vi "move picture.vi"(0 "Picture in":picture, 3 "move":cluster{"x":i16, "y":i16}) -> (14 "Picture out":picture)   [LabVIEW 2019]
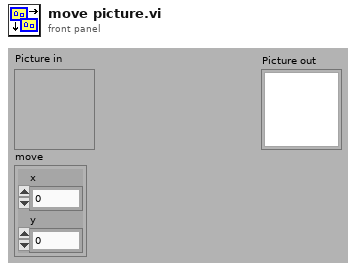
[diagram p1: front panel]
types:
  T1 = typedef "picture op-code.ctl" = u16
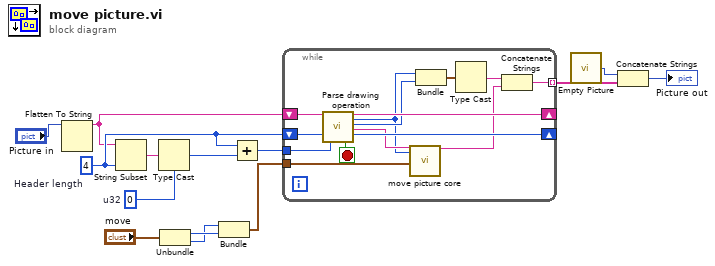
[diagram p0: block diagram]
diagram:
  w5 = u32 0  # u32
  w13 = 4  # Header length
  n1 = Flatten To String(anything="Picture in") -> (data string=w7:string)  [unwired: 3 in, 2 out]
  n2 = String Subset(string=w7, length (rest)=w13) -> (substring=w6:string)  [unwired: 1 in]
  n3 = Type Cast(type=w5, x=w6) -> (*(type *) &x=w14:u32)
  n4 = Unbundle("move") -> ("x"=w3:i16, "y"=w2:i16)
  n5 = Bundle("y"=w2, "x"=w3) -> (w1:cluster{"y":i16, "x":i16})  [unwired: 1 in]
  n6 = Add(x=w13, y=w14) -> (x+y=w12:u32)
  n7 = while {
    shift-right: [w23] -> _
    shift-left: w7 -> [w27]
    shift-right: [w26] -> _
    shift-left: w13 -> [w28]
    tunnel: w12 -> [w24]
    tunnel: [w18] -> w9 mode=indexing
    tunnel: w1 -> [w15]
    stop <- w25 stop-if-true
    n8 = call "Parse drawing operation.vi"("picture data in"=w27, "offset"=w28, "picture size"=w24) -> ("last element"=w25:bool, "picture data out"=w23:string, "op-code"=w16:T1, "data length"=w22:u32, "data string"=w17:string, "offset past element"=w26:i32)  [unwired: 11 in]
    n9 = call "move picture core.vi"("data string in"=w17, "picture op-code"=w16, "move"=w15) -> ("data string out"=w19:string)  [unwired: 16 in]
    n10 = Bundle("op-code"=w16, "data length"=w22) -> (w21:cluster{"op-code":T1, "data length":u32})  [unwired: 1 in]
    n11 = Type Cast(x=w21) -> (*(type *) &x=w20:string)  [unwired: 1 in]
    n12 = Concatenate Strings(w20, w19) -> (w18:string)
  }
  n13 = call "Empty Picture"() -> ("empty picture"=w10:picture)
  n14 = Concatenate Strings(w10, w9) -> (→"Picture out":picture)
